vi "PicoScope2000aSettings.vi"(0 "handle in":i16, 1 "Channel A Settings":T2={"Enabled"=TRUE, "Coupling"=1, "Range"=6, "Analogue Offset"=0.0} {"Analogue Offset" format="%#_6p"; "Range" items=["20 mV"=1, "50 mV"=2, "100 mV"=3, "200 mV"=4, "500 mV"=5, "1 V"=6, "2 V"=7, "5 V"=8, "10 V"=9, "20 V"=10]; "Coupling" items=["AC", "DC"]}, 2 "Channel B Settings":T2={"Enabled"=FALSE, "Coupling"=1, "Range"=6, "Analogue Offset"=0.0} {"Range" items=["20 mV"=1, "50 mV"=2, "100 mV"=3, "200 mV"=4, "500 mV"=5, "1 V"=6, "2 V"=7, "5 V"=8, "10 V"=9, "20 V"=10]; "Coupling" items=["AC", "DC"]}, 3 "Channel C Settings":T2={"Enabled"=FALSE, "Coupling"=1, "Range"=6, "Analogue Offset"=0.0} {"Analogue Offset" format="%#_6p"; "Range" items=["20 mV"=1, "50 mV"=2, "100 mV"=3, "200 mV"=4, "500 mV"=5, "1 V"=6, "2 V"=7, "5 V"=8, "10 V"=9, "20 V"=10]; "Coupling" items=["AC", "DC"]}, 5 "Max_adc":i16=32767, 7 "Device Info":T1, 9 "Trigger Settings":T4={"Trigger Enabled"=FALSE, "Trigger Source"=enum."Channel A", "Trigger Threshold (Volts)"=0.0, "Trigger Direction"=2, "Trigger Delay (samples)"=0, "Auto Trigger Time (ms)"=1000} {"Trigger Direction" items=["Rising"=2, "Falling"=3]}, 11 "error in":errorcluster, 12 "Channel D Settings":T2={"Enabled"=FALSE, "Coupling"=1, "Range"=6, "Analogue Offset"=0.0} {"Analogue Offset" format="%#_6p"; "Range" items=["20 mV"=1, "50 mV"=2, "100 mV"=3, "200 mV"=4, "500 mV"=5, "1 V"=6, "2 V"=7, "5 V"=8, "10 V"=9, "20 V"=10]; "Coupling" items=["AC", "DC"]}, 13 "Port 0 Settings":T3={"Enabled"=FALSE, "Logic Level"=9830} {"Logic Level" items=["1.5V TTL"=9830, "2.5V CMOS"=16383]}, 14 "Port 1 Settings":T3={"Enabled"=FALSE, "Logic Level"=9830} {"Logic Level" items=["1.5V TTL"=9830, "2.5V CMOS"=16383]}) -> (4 "handle out":i16, 8 "Enabled Array":i16[](array[numeric]), 15 "error out":errorcluster)   [LabVIEW 2010]
doc: "This VI is used to set up the oscilloscope. The inputs are clusters for setting channel and simple trigger settings. Advanced triggers can be set up using PicoScope3000aAdvancedTriggerSettings.vi"
uses:
  ps2000a.dll
  PicoScope2000aAnalogChannelSettings.ctl
  PicoScope2000aDigitalChannelSettings.ctl
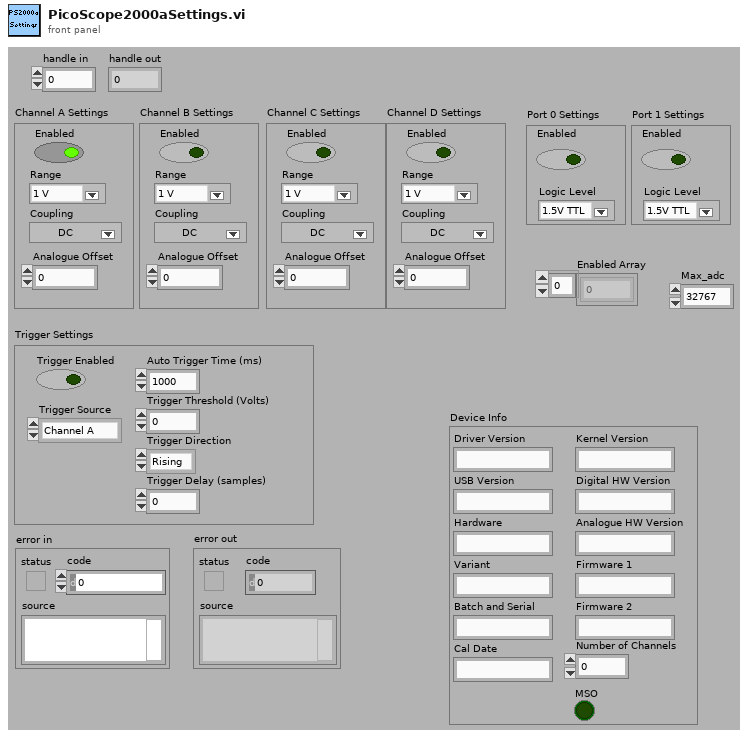
[diagram p1: front panel]
types:
  T1 = cluster{"Driver Version":string, "USB Version":string, "Hardware":string, "Variant":string, "Batch and Serial":string, "Cal Date":string, "Kernel Version":string, "Digital HW Version":string, "Analogue HW Version":string, "Firmware 1":string, "Firmware 2":string, "MSO":bool, "Number of Channels":i16}
  T2 = typedef "PicoScope2000aAnalogChannelSettings.ctl" = cluster{"Enabled":bool, "Coupling":i16, "Range":u32, "Analogue Offset":sgl}
  T3 = typedef "PicoScope2000aDigitalChannelSettings.ctl" = cluster{"Enabled":bool, "Logic Level":i16}
  T4 = cluster{"Trigger Enabled":bool, "Trigger Source":enum16{"Channel A", "Channel B", "Channel C", "Channel D", "Ext."}, "Trigger Threshold (Volts)":dbl, "Trigger Direction":u16, "Trigger Delay (samples)":u32, "Auto Trigger Time (ms)":i16}
  T5 = cluster{"status":bool, "code":u32, "source":string}
  T6 = enum16{"Channel A", "Channel B", "Channel C", "Channel D", "Ext."}
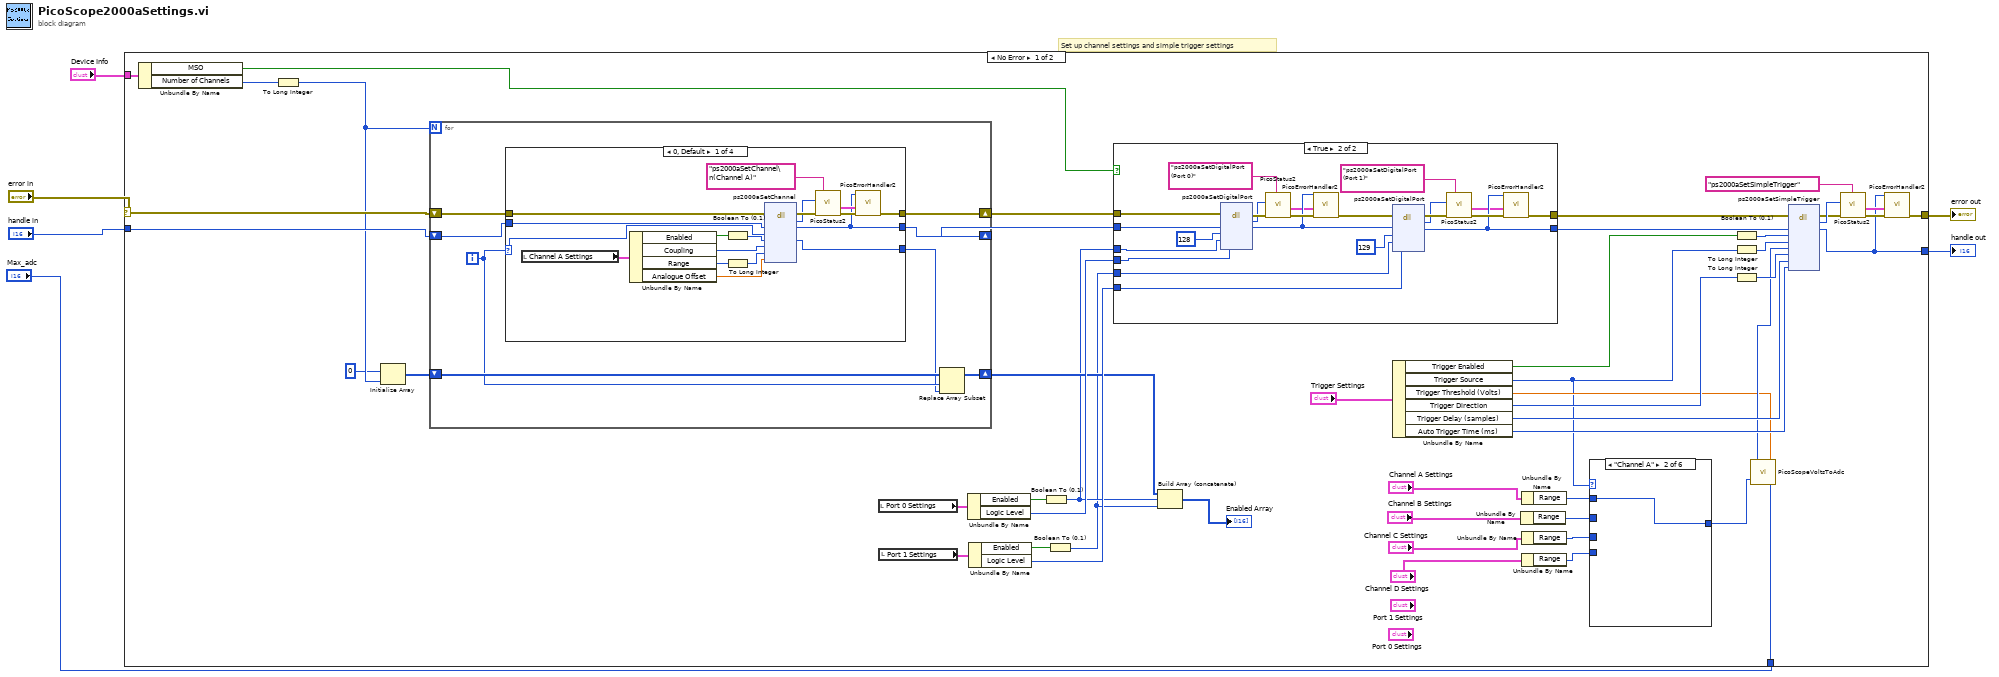
[diagram p0: block diagram]
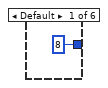
[diagram p2: hidden frame]
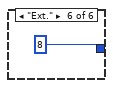
[diagram p6: hidden frame]
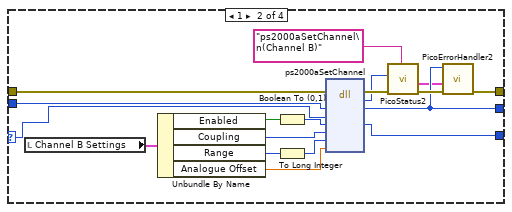
[diagram p8: hidden frame]
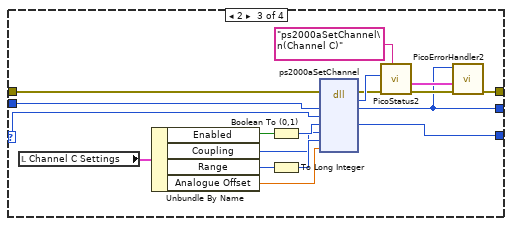
[diagram p9: hidden frame]
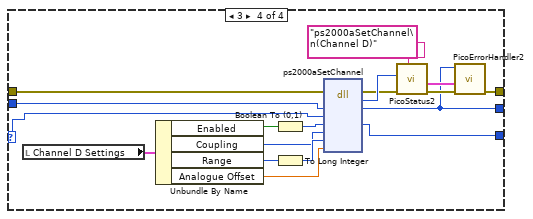
[diagram p10: hidden frame]
diagram:
  # "Set up channel settings and simple trigger settings"
  n1 = case shown="No Error" "error in" {
    selector: "error in" -> [w33 w167]
    tunnel: "handle in" -> [w32 w168]
    tunnel: [w7 w168] -> w2
    tunnel: "Max_adc" -> [w27 _]
    tunnel: "Device Info" -> [w16 _]
    tunnel: [w9 w167] -> w1
    frame No Error {
      n2 = Unbundle By Name(w16) -> ("MSO"=w15:bool, "Number of Channels"=w14:i16)
      n3 = To Long Integer(number=w14) -> (32bit integer=w12:i32)
      n4 = Initialize Array(i16 0 ("element"), w12) -> (w13:i16[])
      n5 = for {
        N: w12 -> [_]
        shift-right: [w94] -> w35
        shift-left: w33 -> [w93]
        shift-right: [w92] -> w34
        shift-left: w32 -> [w91]
        shift-right: [w87] -> w30
        shift-left: w13 -> [w90]
        i -> [w89]
        n6 = case shown="0, Default" w89 {
          selector: w89 -> [w100 w118 w136 w154]
          tunnel: [w97 w116 w134 w152] -> w94
          tunnel: w93 -> [w109 w127 w138 w156]
          tunnel: w91 -> [w108 w126 w137 w155]
          tunnel: [w95 w114 w131 w149] -> w92
          tunnel: [w99 w117 w135 w153] -> w88
          frame 0, Default {
            n7 = local read "Channel A Settings"() -> (w101:T2)
            n8 = Unbundle By Name(w101) -> ("Enabled"=w104:bool, "Coupling"=w107:i16, "Range"=w102:u32, "Analogue Offset"=w106:sgl)
            n9 = Boolean To (0,1)(Boolean=w104) -> (0, 1=w105:i16)
            n10 = To Long Integer(number=w102) -> (32bit integer=w103:i32)
            n11 = dll-call lib="ps2000a.dll" fn="ps2000aSetChannel" ("ps2000a.dll:_ps3000_open_unit@0")(error in=w109, "handle"=w108, "channel"=w100, "enabled"=w105, "dc"=w107, "range"=w103, "analogueOffset"=w106) -> (error out=w111:errorcluster, "PICO_STATUS"=w110:u32, "handle"=w95:i16, "enabled"=w99:i16)  [unwired: 6 in, 1 out]
            n12 = call "PicoStatus2.vi"("PICO source"="ps2000aSetChannel\n(Channel A)" ("source"), "Error in"=w111, "PICO STATUS"=w110) -> ("error out"=w98:errorcluster, "PICO_STATUS out"=w96:T5)  [unwired: 5 in]
            n13 = call "PicoErrorHandler2.vi"("error in (no error)"=w98, "PICO_STATUS in"=w96, "handle In"=w95) -> ("error out"=w97:errorcluster)  [unwired: 8 in]
          }
          frame 1 {
            n14 = local read "Channel B Settings"() -> (w119:T2)
            n15 = Unbundle By Name(w119) -> ("Enabled"=w122:bool, "Coupling"=w125:i16, "Range"=w120:u32, "Analogue Offset"=w124:sgl)
            n16 = Boolean To (0,1)(Boolean=w122) -> (0, 1=w123:i16)
            n17 = To Long Integer(number=w120) -> (32bit integer=w121:i32)
            n18 = dll-call lib="ps2000a.dll" fn="ps2000aSetChannel" ("ps2000a.dll:_ps3000_open_unit@0")(error in=w127, "handle"=w126, "channel"=w118, "enabled"=w123, "dc"=w125, "range"=w121, "analogueOffset"=w124) -> (error out=w129:errorcluster, "PICO_STATUS"=w128:u32, "handle"=w114:i16, "enabled"=w117:i16)  [unwired: 6 in, 1 out]
            n19 = call "PicoStatus2.vi"("PICO source"="ps2000aSetChannel\n(Channel B)" ("source"), "Error in"=w129, "PICO STATUS"=w128) -> ("error out"=w115:errorcluster, "PICO_STATUS out"=w113:T5)  [unwired: 5 in]
            n20 = call "PicoErrorHandler2.vi"("error in (no error)"=w115, "PICO_STATUS in"=w113, "handle In"=w114) -> ("error out"=w116:errorcluster)  [unwired: 8 in]
          }
          frame 2 {
            n21 = local read "Channel C Settings"() -> (w148:T2)
            n22 = Unbundle By Name(w148) -> ("Enabled"=w145:bool, "Coupling"=w142:i16, "Range"=w147:u32, "Analogue Offset"=w143:sgl)
            n23 = Boolean To (0,1)(Boolean=w145) -> (0, 1=w144:i16)
            n24 = To Long Integer(number=w147) -> (32bit integer=w146:i32)
            n25 = dll-call lib="ps2000a.dll" fn="ps2000aSetChannel" ("ps2000a.dll:_ps3000_open_unit@0")(error in=w138, "handle"=w137, "channel"=w136, "enabled"=w144, "dc"=w142, "range"=w146, "analogueOffset"=w143) -> (error out=w140:errorcluster, "PICO_STATUS"=w141:u32, "handle"=w131:i16, "enabled"=w135:i16)  [unwired: 6 in, 1 out]
            n26 = call "PicoStatus2.vi"("PICO source"="ps2000aSetChannel\n(Channel C)" ("source"), "Error in"=w140, "PICO STATUS"=w141) -> ("error out"=w133:errorcluster, "PICO_STATUS out"=w132:T5)  [unwired: 5 in]
            n27 = call "PicoErrorHandler2.vi"("error in (no error)"=w133, "PICO_STATUS in"=w132, "handle In"=w131) -> ("error out"=w134:errorcluster)  [unwired: 8 in]
          }
          frame 3 {
            n28 = local read "Channel D Settings"() -> (w166:T2)
            n29 = Unbundle By Name(w166) -> ("Enabled"=w163:bool, "Coupling"=w160:i16, "Range"=w165:u32, "Analogue Offset"=w161:sgl)
            n30 = Boolean To (0,1)(Boolean=w163) -> (0, 1=w162:i16)
            n31 = To Long Integer(number=w165) -> (32bit integer=w164:i32)
            n32 = dll-call lib="ps2000a.dll" fn="ps2000aSetChannel" ("ps2000a.dll:_ps3000_open_unit@0")(error in=w156, "handle"=w155, "channel"=w154, "enabled"=w162, "dc"=w160, "range"=w164, "analogueOffset"=w161) -> (error out=w158:errorcluster, "PICO_STATUS"=w159:u32, "handle"=w149:i16, "enabled"=w153:i16)  [unwired: 6 in, 1 out]
            n33 = call "PicoStatus2.vi"("PICO source"="ps2000aSetChannel\n(Channel D)" ("source"), "Error in"=w158, "PICO STATUS"=w159) -> ("error out"=w151:errorcluster, "PICO_STATUS out"=w150:T5)  [unwired: 5 in]
            n34 = call "PicoErrorHandler2.vi"("error in (no error)"=w151, "PICO_STATUS in"=w150, "handle In"=w149) -> ("error out"=w152:errorcluster)  [unwired: 8 in]
          }
        }
        n35 = Replace Array Subset(array=w90, new element=w88, index=w89) -> (w87:i16[])
      }
      n36 = local read "Port 0 Settings"() -> (w42:T3)
      n37 = local read "Port 1 Settings"() -> (w40:T3)
      n38 = Unbundle By Name(w42) -> ("Enabled"=w43:bool, "Logic Level"=w39:i16)
      n39 = Unbundle By Name(w40) -> ("Enabled"=w41:bool, "Logic Level"=w38:i16)
      n40 = Boolean To (0,1)(Boolean=w43) -> (0, 1=w29:i16)
      n41 = Boolean To (0,1)(Boolean=w41) -> (0, 1=w28:i16)
      n42 = case shown="True" w15 {
        tunnel: w29 -> [_ w78]
        tunnel: w39 -> [_ w77]
        tunnel: w28 -> [_ w76]
        tunnel: w38 -> [_ w75]
        tunnel: [w64 w67] -> w37
        tunnel: [w63 w66] -> w36
        tunnel: w35 -> [w64 w74]
        tunnel: w34 -> [w63 w73]
        frame False {
        }
        frame True {
          n43 = dll-call lib="PS2000a.dll" fn="ps2000aSetDigitalPort"(error in=w74, "handle"=w73, "port"=u32 128 ("channel"), "enabled"=w78, "logicLevel"=w77) -> (error out=w86:errorcluster, "PICO_STATUS"=w84:u32, "handle"=w71:i16)  [unwired: 5 in, 1 out]
          n44 = call "PicoStatus2.vi"("PICO source"="ps2000aSetDigitalPort (Port 0)" ("source"), "Error in"=w86, "PICO STATUS"=w84) -> ("error out"=w72:errorcluster, "PICO_STATUS out"=w69:T5)  [unwired: 5 in]
          n45 = call "PicoErrorHandler2.vi"("error in (no error)"=w72, "PICO_STATUS in"=w69, "handle In"=w71) -> ("error out"=w70:errorcluster)  [unwired: 8 in]
          n46 = dll-call lib="PS2000a.dll" fn="ps2000aSetDigitalPort"(error in=w70, "handle"=w71, "port"=u32 129 ("channel"), "enabled"=w76, "logicLevel"=w75) -> (error out=w82:errorcluster, "PICO_STATUS"=w80:u32, "handle"=w66:i16)  [unwired: 5 in, 1 out]
          n47 = call "PicoStatus2.vi"("PICO source"="ps2000aSetDigitalPort (Port 1)" ("source"), "Error in"=w82, "PICO STATUS"=w80) -> ("error out"=w68:errorcluster, "PICO_STATUS out"=w65:T5)  [unwired: 5 in]
          n48 = call "PicoErrorHandler2.vi"("error in (no error)"=w68, "PICO_STATUS in"=w65, "handle In"=w66) -> ("error out"=w67:errorcluster)  [unwired: 8 in]
        }
      }
      n49 = Build Array (concatenate)(w30, w29, w28) -> (→"Enabled Array":i16[])
      n50 = Unbundle By Name("Trigger Settings") -> ("Trigger Enabled"=w50:bool, "Trigger Source"=w25:T6, "Trigger Threshold (Volts)"=w44:dbl, "Trigger Direction"=w53:u16, "Trigger Delay (samples)"=w52:u32, "Auto Trigger Time (ms)"=w51:i16)
      n51 = Unbundle By Name("Channel B Settings") -> ("Range"=w23:u32)
      n52 = Unbundle By Name("Channel A Settings") -> ("Range"=w24:u32)
      n53 = Unbundle By Name("Channel C Settings") -> ("Range"=w22:u32)
      n54 = Unbundle By Name("Channel D Settings") -> ("Range"=w21:u32)
      n55 = case shown="\"Channel A\"" w25 {
        tunnel: [u16 8 ("Range") w58 w59 w60 w61 u16 8 ("Range")] -> w26
        tunnel: w24 -> [_ w58 _ _ _ _]
        tunnel: w23 -> [_ _ w59 _ _ _]
        tunnel: w22 -> [_ _ _ w60 _ _]
        tunnel: w21 -> [_ _ _ _ w61 _]
        frame Default {
        }
        frame "Channel A" {
        }
        frame "Channel B" {
        }
        frame "Channel C" {
        }
        frame "Channel D" {
        }
        frame "Ext." {
        }
      }
      n56 = Boolean To (0,1)(Boolean=w50) -> (0, 1=w49:i16)
      n57 = To Long Integer(number=w25) -> (32bit integer=w56:i32)
      n58 = To Long Integer(number=w53) -> (32bit integer=w55:i32)
      n59 = call "PicoScopeVoltsToAdc.vi"("Max_adc"=w27, "Units"=w44, "Range Index"=w26) -> ("ADC count"=w45:i16)
      n60 = dll-call lib="ps2000a.dll" fn="ps2000aSetSimpleTrigger" ("ps2000a.dll:_ps3000_open_unit@0")(error in=w37, "handle"=w36, "enabled"=w49, "source"=w56, "threshold"=w45, "direction"=w55, "delay"=w52, "autoTrigger_ms"=w51) -> (error out=w47:errorcluster, "PICO_STATUS"=w48:u32, "handle"=w7:i16)  [unwired: 8 in, 1 out]
      n61 = call "PicoStatus2.vi"("PICO source"="ps2000aSetSimpleTrigger" ("source"), "Error in"=w47, "PICO STATUS"=w48) -> ("error out"=w10:errorcluster, "PICO_STATUS out"=w8:T5)  [unwired: 5 in]
      n62 = call "PicoErrorHandler2.vi"("error in (no error)"=w10, "PICO_STATUS in"=w8, "handle In"=w7) -> ("error out"=w9:errorcluster)  [unwired: 8 in]
    }
    frame Error {
    }
  }
  "handle out" <- w2
  "error out" <- w1
